vi "Get first unused item.vi"(8 "error in (no error)":errorcluster, 11 "Pool":T1[](array[typedef])=[{"index"=0, "state"=enum."unused"}, {"index"=1, "state"=enum."unused"}, {"index"=2, "state"=enum."unused"}, {"index"=3, "state"=enum."unused"}, {"index"=4, "state"=enum."unused"}, {"index"=5, "state"=enum."unused"}]) -> (0 "error out":errorcluster, 1 "index of first unused item":i32, 2 "T = unused item was found":bool, 3 "First unused item":T1)   [LabVIEW 2021, in "Numeric Utilities.lvlib"]
uses:
  Numeric Utilities.lvlib
  cluster-touched index.ctl
  index state enum.ctl
panel:
  # "Development\ncontrols/indicators useful for development and testing, but which are not outputs of the VI"
  # "Input\nInputs to the VI"
  # "Output\nOutputs of the VI"
  # "Description\n\nBlank VI with error handling case. \n\nSummarize the use of this VI in this space."
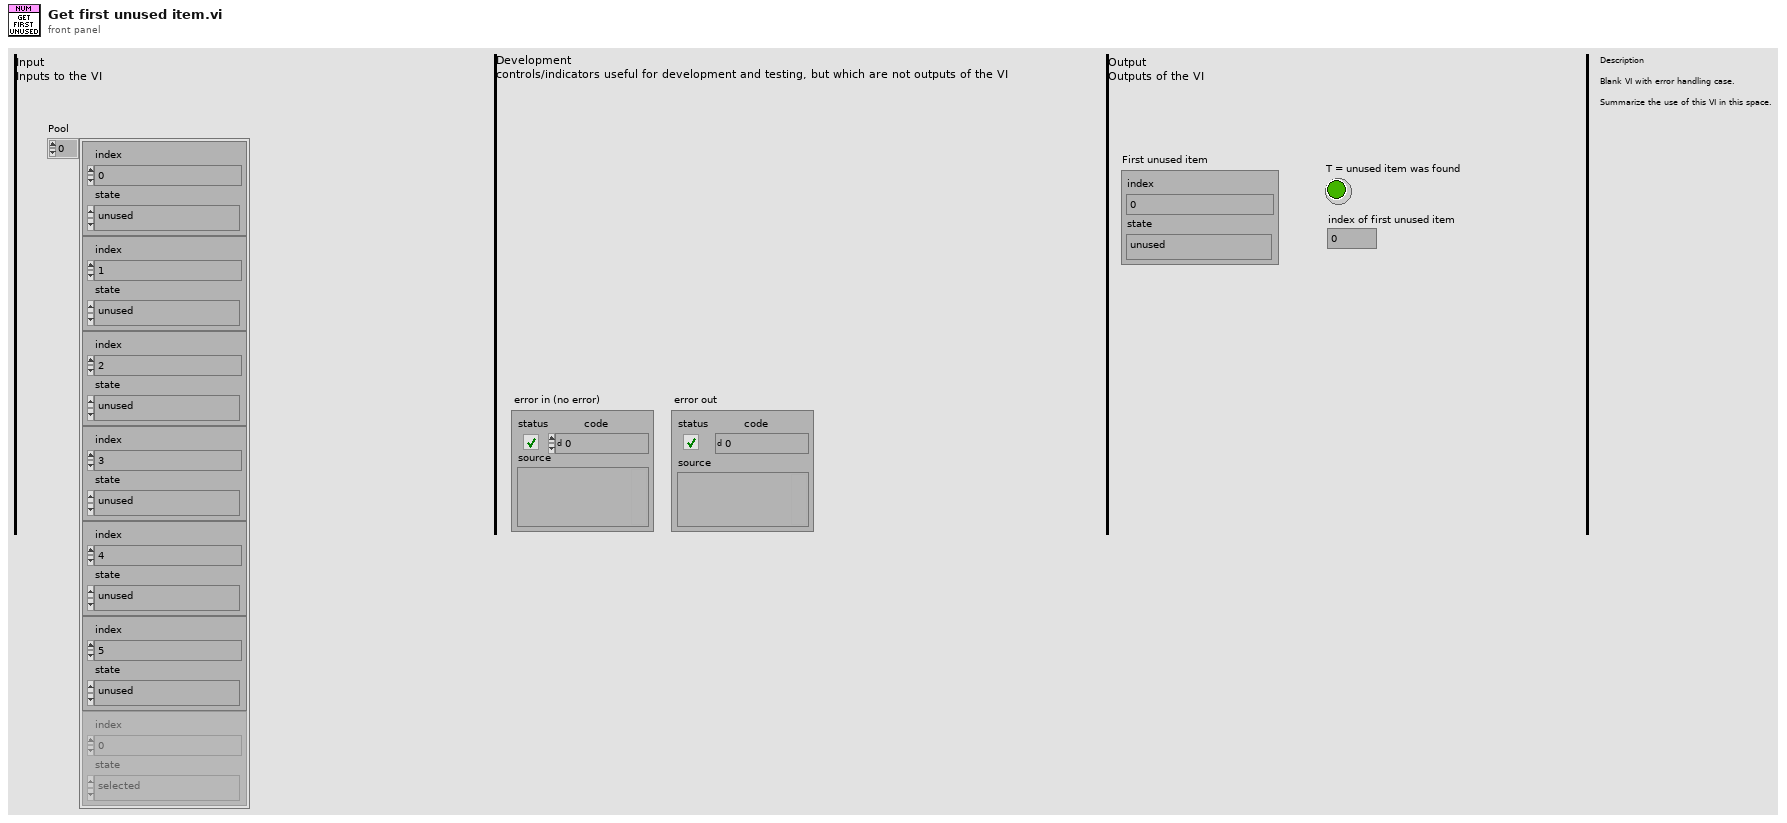
[diagram p1: front panel]
types:
  T1 = typedef "Numeric Utilities.lvlib/cluster-touched index.ctl" = cluster{"index":i32, "state":T2}
  T2 = typedef "Numeric Utilities.lvlib/index state enum.ctl" = enum16{"unused", "selected", "exhausted"}
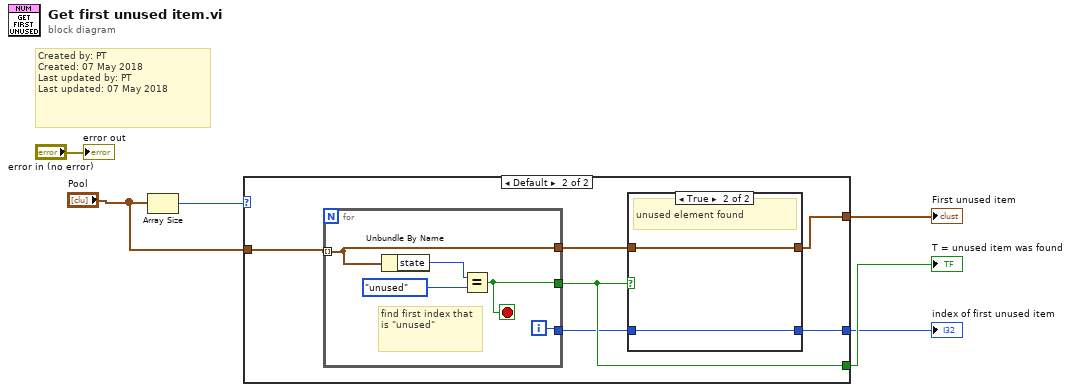
[diagram p0: block diagram]
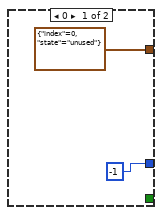
[diagram p2: hidden frame]
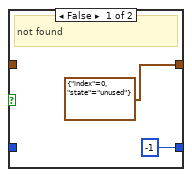
[diagram p3: hidden frame]
diagram:
  # "Created by: PT\nCreated: 07 May 2018\nLast updated by: PT\nLast updated: 07 May 2018"
  n1 = Array Size(array="Pool") -> (size(s)=w4:i32)
  n2 = case shown="Default" w4 {
    tunnel: "Pool" -> [_ w14]
    tunnel: [_ w13] -> w3
    tunnel: [T1 {"index"=0, "state"=enum."unused"} w11] -> w2
    tunnel: [-1 w9] -> w1
    frame 0 {
    }
    frame Default {
      n3 = for {
        tunnel: w14 -> [w20] mode=indexing
        tunnel: [w21] -> w13
        tunnel: [w20] -> w12
        tunnel: [w19] -> w10
        i -> [w19]
        stop <- w21 stop-if-true
        # "find first index that is \"unused\""
        n4 = Unbundle By Name(w20) -> ("state"=w23:T2)
        n5 = Equal?(x=w23, y=index_state_enum."unused") -> (x = y?=w21:bool)
      }
      n6 = case shown="True" w13 {
        tunnel: w12 -> [_ w18]
        tunnel: [T1 {"index"=0, "state"=enum."unused"} w18] -> w11
        tunnel: w10 -> [_ w17]
        tunnel: [-1 w17] -> w9
        frame False {
          # "not found"
        }
        frame True {
          # "unused element found"
        }
      }
    }
  }
  "T = unused item was found" <- w3
  "First unused item" <- w2
  "index of first unused item" <- w1
  "error out" <- "error in (no error)"
